vi "ELVIS III v1.0 Close DI Block.vi"(8 "error in (no error)":errorcluster, 10 "DI (N Samples) Channel List":T3, 11 "myRIO Ref In":T1) -> (0 "error out":errorcluster)   [LabVIEW 2021]
uses:
  <vilib>/myRIO/Common/Instrument Driver Framework/myRIO v1.0/DI Block/typedefs/DI Block Channels List.ctl
  <vilib>/myRIO/Common/Instrument Driver Framework/myRIO v1.0/DI Block/typedefs/DI Block Channels Enum.ctl
  <vilib>/myRIO/Common/Instrument Driver Framework/Utilities/typedefs/myRIO v1.0 Reference.ctl
  <vilib>/myRIO/Common/Instrument Driver Framework/Utilities/typedefs/Generic FPGA Reference.ctl
  <vilib>/myRIO/Common/Instrument Driver Framework/ELVIS III v1.0/DI Block/vis/ELVIS III v1.0 Build MUX Configuration DI Block.vi
  <vilib>/myRIO/Common/Instrument Driver Framework/ELVIS III v1.0/Resource Manager/vis/ELVIS III v1.0 Create Configuration List.vi
  <vilib>/myRIO/Common/Instrument Driver Framework/ELVIS III v1.0/Resource Manager/vis/ELVIS III v1.0 Configure IO.vi
  <vilib>/myRIO/Common/Instrument Driver Framework/ELVIS III v1.0/Resource Manager/vis/ELVIS III v1.0 Configure DI Mode.vi
  <vilib>/myRIO/Common/Instrument Driver Framework/ELVIS III v1.0/Resource Manager/vis/ELVIS III v1.0 Unreserve Channel List.vi
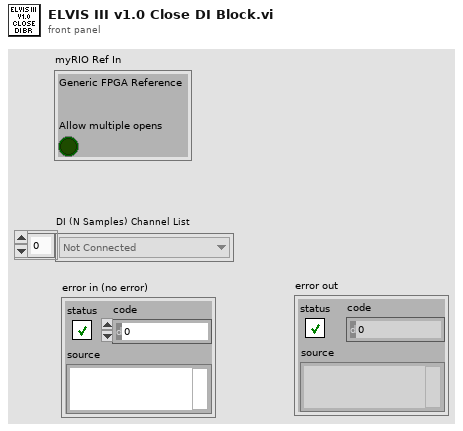
[diagram p1: front panel]
types:
  T1 = typedef "myRIO v1.0 Reference.ctl" = cluster{"Generic FPGA Reference":T2, "Allow multiple opens":bool}
  T2 = typedef "Generic FPGA Reference.ctl" = refnum<k20>
  T3 = typedef "DI Block Channels List.ctl" = T4[]
  T4 = typedef "DI Block Channels Enum.ctl" = enum16{"Not Connected", "A/DI0 (N Samples)", "A/DI1 (N Samples)", "A/DI2 (N Samples)", "A/DI3 (N Samples)", "A/DI4 (N Samples)", "A/DI5 (N Samples)", "A/DI6 (N Samples)", "A/DI7 (N Samples)", "A/DI8 (N Samples)", "A/DI9 (N Samples)", "A/DI10 (N Samples)", "A/DI11 (N Samples)", "A/DI12 (N Samples)", "A/DI13 (N Samples)", "A/DI14 (N Samples)", "A/DI15 (N Samples)", "A/DI16 (N Samples)", "A/DI17 (N Samples)", "A/DI18 (N Samples)", "A/DI19 (N Samples)", "B/DI0 (N Samples)", "B/DI1 (N Samples)", "B/DI2 (N Samples)", "B/DI3 (N Samples)", "B/DI4 (N Samples)", "B/DI5 (N Samples)", "B/DI6 (N Samples)", "B/DI7 (N Samples)", "B/DI8 (N Samples)", "B/DI9 (N Samples)", "B/DI10 (N Samples)", "B/DI11 (N Samples)", "B/DI12 (N Samples)", "B/DI13 (N Samples)", "B/DI14 (N Samples)", "B/DI15 (N Samples)", "B/DI16 (N Samples)", "B/DI17 (N Samples)", "B/DI18 (N Samples)", "B/DI19 (N Samples)"}
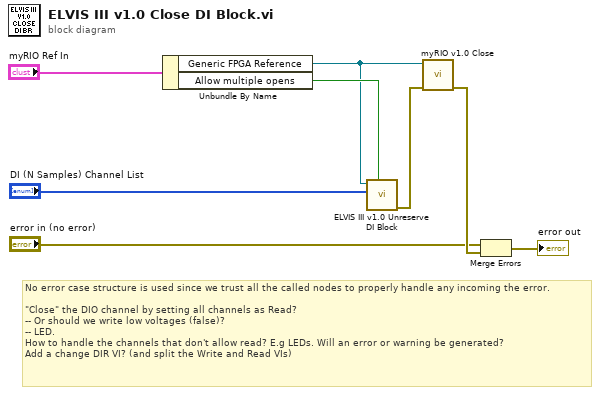
[diagram p0: block diagram]
diagram:
  # "No error case structure is used since we trust all the called nodes to properly handle any incoming the error.\n\n\"Close\" the DIO channel by setting all channels as Read?\n-- Or should we write low voltages (false)?\n-- LED.\nHow to handle the channels that don't allow read? E.g LEDs. Will an error or warning be generated?\nAdd a change DIR VI? (and split the Write and Read VIs)"
  n1 = Unbundle By Name("myRIO Ref In") -> ("Generic FPGA Reference"=w1:T2, "Allow multiple opens"=w6:bool)
  n2 = call <vilib>:"ELVIS III v1.0 Unreserve DI Block.vi"("Allow multiple opens?"=w6, "DI (N Samples) Channel List"="DI (N Samples) Channel List", "Generic FPGA Reference"=w1) -> ("error out"=w8:errorcluster)  [unwired: 8 in]
  n3 = call <vilib>:"myRIO v1.0 Close.vi"("error in (no error)"=w8, "myRIO FPGA Ref In"=w1) -> ("error out"=w7:errorcluster)  [unwired: 9 in]
  n4 = Merge Errors("error in (no error)", w7) -> (→"error out":errorcluster)
